vi "format data.vi"(10 "Temp Array":dbl[][](array[numeric]), 11 "Time Array":timestamp[][](array[timestamp])) -> (3 "Array":string[][](array[string]))   [LabVIEW 2025, in "data log.lvclass"]
uses:
  data log.lvclass
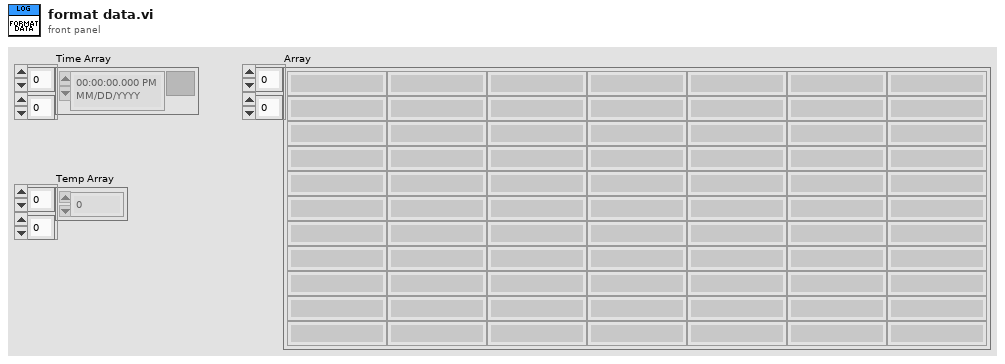
[diagram p1: front panel]
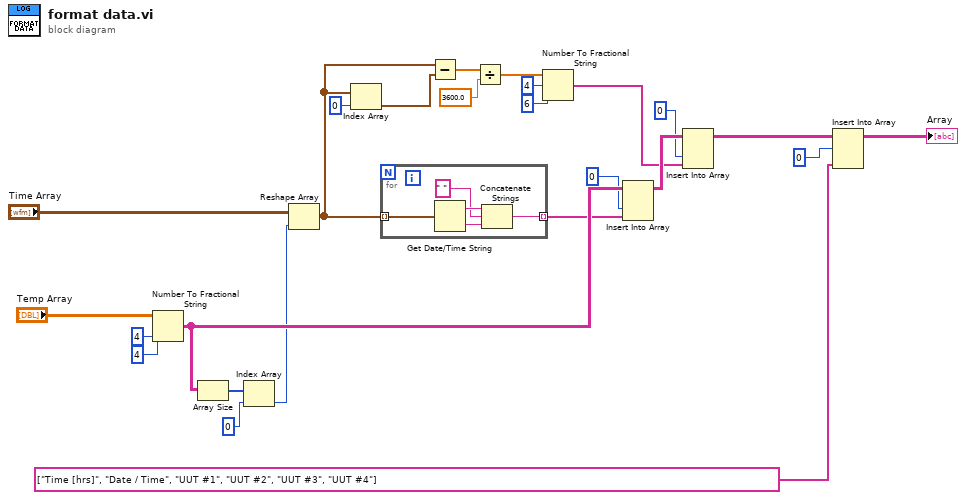
[diagram p0: block diagram]
diagram:
  n1 = Number To Fractional String(number="Temp Array", width (-)=i16 4, precision (6)=i16 4) -> (F-format string=w25:string[][])  [unwired: 1 in]
  n2 = Array Size(array=w25) -> (size(s)=w20:i32[])
  n3 = Index Array(array=w20, index=0) -> (element=w22:i32)
  n4 = Reshape Array("Time Array", w22) -> (w14:timestamp[])
  n5 = Index Array(array=w14, index=0) -> (element=w13:timestamp)
  n6 = for {
    tunnel: w14 -> [w30] mode=indexing
    tunnel: [w28] -> w23 mode=indexing
    n7 = Get Date/Time String(seconds (now)=w30) -> (date string=w27:string, time string=w29:string)  [unwired: 2 in]
    n8 = Concatenate Strings(w27, " ", w29) -> (w28:string)
  }
  n9 = Subtract(x=w14, y=w13) -> (x-y=w12:dbl[])
  n10 = Divide(x=w12, y=3600.0) -> (x/y=w10:dbl[])
  n11 = Number To Fractional String(number=w10, width (-)=i16 4, precision (6)=i16 6) -> (F-format string=w6:string[])  [unwired: 1 in]
  n12 = Insert Into Array(array=w25, index (col)=0 ("index (row)"), new element=w23) -> (w7:string[][])  [unwired: 1 in]
  n13 = Insert Into Array(array=w7, index (col)=0 ("disabled index (col)"), new element=w6) -> (w4:string[][])  [unwired: 1 in]
  n14 = Insert Into Array(array=w4, index (row)=0, new element=string[] ["Time [hrs]", "Date / Time", "UUT #1", "UUT #2", "UUT #3", "UUT #4"]) -> (→"Array":string[][])  [unwired: 1 in]
